vi "Transmit.vi"(6 "Data Input(Hex)":string="11223344556677 88", 8 "错误输入（无错误）":errorcluster, 9 "ID(Hex 高位有效)":string="80000000", 10 "CANChannel":u32, 11 "DeviceType":T3=3 items=["PCI-CAN200"=7, "USB-CAN"=2, "USB-CAN200"=3]) -> (0 "错误输出":errorcluster, 2 "Result":bool, 3 "DeviceTypeOut":u16(ring)=7 items=["PCI-CAN200"=7])   [LabVIEW 2013]
uses:
  DevType.ctl
  VCI_CAN.dll
panel:
  out "十六进制整型字符串":string
  out "pSend":T1 {"ID" format="%02x"; "ID2" format="%02x"; "ID1" format="%02x"; "ID0" format="%02x"}
  out "VCI_CAN_OBJ_T":T2={"ID"=0, "ID2"=0, "ID1"=0, "ID0"=0, "TimeStamp"=0, "TimeFlag"=0, "SendType"=1, "RemoteFlag"=0, "ExternFlag"=0, "DataLen"=8, 0, 0, 0, 0, 0, 0, 0, 0, 0, 0, 0} {"ID0" format="%x"; "ID1" format="%x"; "ID2" format="%x"; "?" format="%02x"; "?" format="%02x"; "?" format="%02x"; "?" format="%02x"; "?" format="%02x"; "?" format="%02x"; "?" format="%02x"; "?" format="%02x"; "ID" format="%x"}
  out "Frame Format":u8(ring) items=["Data Frame", "Remote Frame"]
  out "Frame Type":u8(ring) items=["Standard Frame", "Extend Frame"]
  out "Transmit Type":u8(ring) items=["Normal Transmit"]
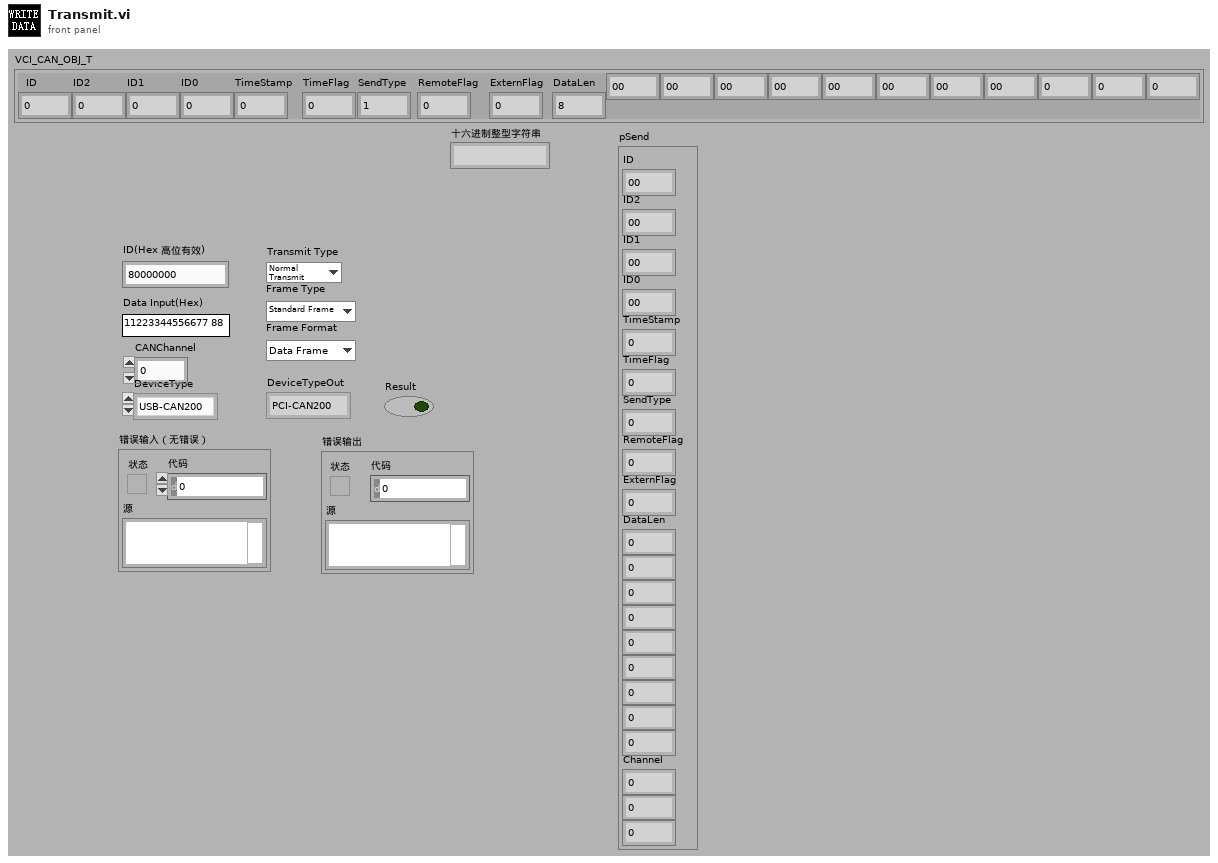
[diagram p1: front panel]
types:
  T1 = cluster{"ID":u8, "ID2":u8, "ID1":u8, "ID0":u8, "TimeStamp":u32, "TimeFlag":u8, "SendType":u8, "RemoteFlag":u8, "ExternFlag":u8, "DataLen":u8, u8, u8, u8, u8, u8, u8, u8, u8, "Channel":u8, u8, u8}
  T2 = cluster{"ID":u8, "ID2":u8, "ID1":u8, "ID0":u8, "TimeStamp":u32, "TimeFlag":u8, "SendType":u8, "RemoteFlag":u8, "ExternFlag":u8, "DataLen":u8, u8, u8, u8, u8, u8, u8, u8, u8, u8, u8, u8}
  T3 = typedef "DevType.ctl" = u16
  T4 = cluster{"Transmit Type":u8, "Frame Type":u8, "Frame Format":u8, "Data Input(Hex)":string, "ID(Hex 高位有效)":string}
  T5 = cluster{"[0]":u8, "[1]":u8, "[2]":u8, "[3]":u8, "[4]":u8, "[5]":u8, "[6]":u8, "[7]":u8, "[8]":u8}
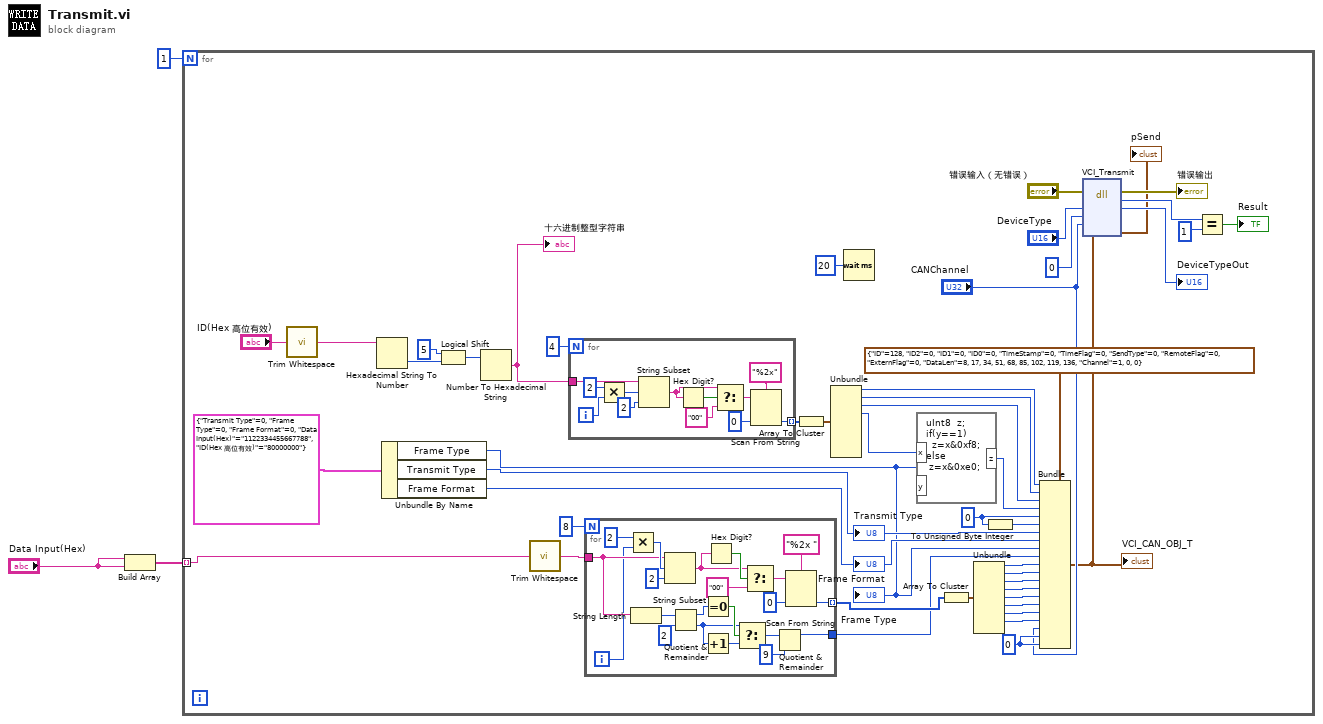
[diagram p0: block diagram]
diagram:
  n1 = Build Array("Data Input(Hex)", "Data Input(Hex)") -> (w2:string[])
  n2 = for {
    N: 1 -> [_]
    tunnel: w2 -> [w5] mode=indexing
    w44 = u8 0
    w35 = u32 0
    n3 = call <vilib>:"Trim Whitespace.vi"("string"="ID(Hex 高位有效)") -> ("trimmed string"=w7:string)  [unwired: 1 in]
    n4 = Hexadecimal String To Number(string=w7) -> (number=w10:u32)  [unwired: 2 in, 1 out]
    n5 = Unbundle By Name(T4 {"Transmit Type"=0, "Frame Type"=0, "Frame Format"=0, "Data Input(Hex)"="1122334455667788", "ID(Hex 高位有效)"="80000000"} ("CanParas")) -> ("Frame Type"=w16:u8, "Transmit Type"=w21:u8, "Frame Format"=w20:u8)
    "Transmit Type" <- w21
    "Frame Type" <- w16
    "Frame Format" <- w20
    n6 = Logical Shift(y=i8 5, x=w10) -> (x << y=w8:u32)
    n7 = Number To Hexadecimal String(2:w8) -> (0:w6:string)  [unwired: 1 in]
    "十六进制整型字符串" <- w6
    n8 = call <vilib>:"Trim Whitespace.vi"("string"=w5) -> ("trimmed string"=w12:string)  [unwired: 1 in]
    n9 = for {
      N: 4 -> [_]
      tunnel: w6 -> [w54]
      tunnel: [w53] -> w28 mode=indexing
      i -> [w60]
      n10 = Multiply(x=2, y=w60) -> (x*y=w58:i32)
      n11 = String Subset(string=w54, offset (0)=w58, length (rest)=2) -> (substring=w56:string)
      n12 = Hex Digit?(1:w56) -> (0:w55:bool)
      n13 = Select(t=w56, s=w55, f="00") -> (s? t:f=w57:string)
      n14 = Scan From String(format string="%2x", input string=w57, default 1=u8 0 ("默认值 1")) -> (output 1=w53:u8)  [unwired: 2 in, 3 out]
    }
    n15 = for {
      N: 8 -> [_]
      tunnel: w12 -> [w77]
      tunnel: [w80] -> w33 mode=indexing
      tunnel: [w65] -> w31
      i -> [w70]
      n16 = Multiply(x=2, y=w70) -> (x*y=w83:i32)
      n17 = String Length(string=w77) -> (length=w76:i32)
      n18 = String Subset(string=w77, offset (0)=w83, length (rest)=2 ("length (rest)")) -> (substring=w74:string)
      n19 = Quotient & Remainder(x=w76, y=2) -> (x-y*floor(x/y)=w72:i32, floor(x/y)=w68:i32)
      n20 = Equal To 0?(x=w72) -> (x = 0?=w71:bool)
      n21 = Increment(x=w68) -> (x+1=w69:i32)
      n22 = Hex Digit?(1:w74) -> (0:w78:bool)
      n23 = Select(t=w68, s=w71, f=w69) -> (s? t:f=w67:i32)
      n24 = Select(t=w74, s=w78, f="00" ("t")) -> (s? t:f=w79:string)
      n25 = Quotient & Remainder(x=w67, y=9) -> (x-y*floor(x/y)=w65:i32)  [unwired: 1 out]
      n26 = Scan From String(format string="%2x ", input string=w79, default 1=u8 0 ("默认值 1")) -> (output 1=w80:u8)  [unwired: 2 in, 3 out]
    }
    n27 = Array To Cluster(array=w28) -> (cluster=w27:T5)
    n28 = Unbundle(w27) -> ("[0]"=w26:u8, "[1]"=w25:u8, "[2]"=w24:u8, "[3]"=w15:u8)  [unwired: 5 out]
    n29 = Wait (ms)(milliseconds to wait=u32 20 ("等待时间（毫秒）")) -> ()  [unwired: 1 out]
    n30 = formula code="uInt8  z; \nif(y==1)\n  z=x&0xf8;\nelse\n z=x&0xe0;"("x"=w15, "y"=w16) -> ("z"=w13:u8)
    n31 = Array To Cluster(array=w33) -> (cluster=w32:T5)
    n32 = Unbundle(w32) -> ("[0]"=w36:u8, "[1]"=w37:u8, "[2]"=w38:u8, "[3]"=w39:u8, "[4]"=w40:u8, "[5]"=w41:u8, "[6]"=w42:u8, "[7]"=w43:u8)  [unwired: 1 out]
    n33 = To Unsigned Byte Integer(number=w35) -> (unsigned 8bit integer=w34:u8)
    n34 = Bundle(cluster=T1 {"ID"=128, "ID2"=0, "ID1"=0, "ID0"=0, "TimeStamp"=0, "TimeFlag"=0, "SendType"=0, "RemoteFlag"=0, "ExternFlag"=0, "DataLen"=8, 17, 34, 51, 68, 85, 102, 119, 136, "Channel"=1, 0, 0} ("VCI_CAN_OBJ_T 2"), "ID"=w26, "ID2"=w25, "ID1"=w24, "ID0"=w13, "TimeStamp"=w35, "TimeFlag"=w34, "SendType"=w21, "RemoteFlag"=w20, "ExternFlag"=w16, "DataLen"=w31, w36, w37, w38, w39, w40, w41, w42, w43, "Channel"="CANChannel", w44, w44) -> (w18:T1)
    "VCI_CAN_OBJ_T" <- w18
    n35 = dll-call lib="PTH1abs CUsers\nAdministratorDesktop360æºç åå¤360å¨æ¯ä¸»æºæåæµè¯V816InstrumentDriversUSB-CANVCI_CAN.dll" fn="VCI_Transmit"(error in="错误输入（无错误）", "DeviceType"="DeviceType", "DeviceInd"=0, "CANInd"="CANChannel", "pSend"=w18) -> (error out=→"错误输出":errorcluster, "返回类型"=w47:u32, "DeviceType"=→"DeviceTypeOut":u32, "pSend"=→"pSend":T1)  [unwired: 4 in, 1 out]
    n36 = Equal?(x=w47, y=u32 1) -> (x = y?=→"Result":bool)
  }
